vi "Configure Width Trigger.vi"(0 "VISA resource name":refnum<visa-resource-name>, 1 "Trigger Slope (0: Rising)":u16(ring) items=["Rising", "Falling"], 2 "Trigger Source (0: Channel 1)":u16(ring) items=["Channel 1", "Channel 2", "Channel 3", "Channel 4", "External", "Pattern", "Ext", "Ext10"], 5 "Trigger Level (0.0 V)":dbl, 9 "Mode (0: Less Than)":u16(ring) items=["Less Than", "Greater Than", "In Range/Out Of Range"], 11 "error in (no error)":errorcluster, 12 "Limit 1 (4 ns)":dbl=4e-09, 13 "Limit 2 (6 ns)":dbl=6e-09) -> (4 "VISA resource name out":refnum<visa-resource-name>, 15 "error out":errorcluster)   [LabVIEW 2020, in "LeCroy Wave Series.lvlib"]
doc: "Configures width trigger settings. Width trigger allows you to define a positive- or\nnegative-going pulse width bounded by a voltage level, above or below which a trigger\nwill occur. Or you can specify a pulse width and voltage range, within or outside of\nwhich a trigger will occur.\n\nNote: \"External\" is included for the purpose of backwards compatibility. Use EXT or EXT10 for best results."
uses:
  LeCroy Wave Series.lvlib
panel:
  # "Note: \"External\" is included for the purpose\nof backwards compatibility.  Use EXT or EXT10\nfor best results."
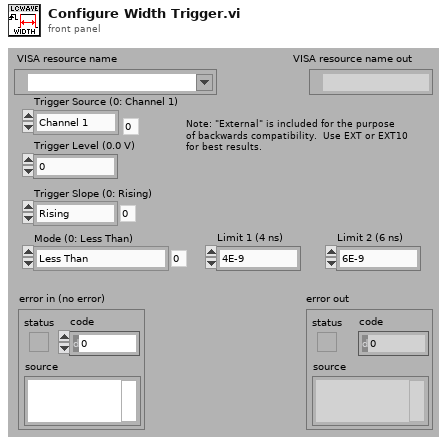
[diagram p1: front panel]
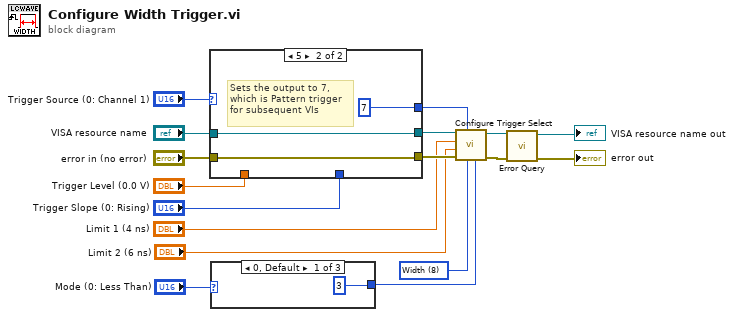
[diagram p0: block diagram]
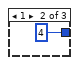
[diagram p2: hidden frame]
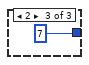
[diagram p3: hidden frame]
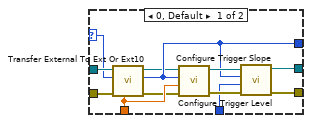
[diagram p4: hidden frame]
diagram:
  w2 = u16 8 items=["Edge", "Dropout", "Glitch", "Interval", "Std", "Sng", "State Qualify", "Edge Qualify", "Width"] ("Trigger type")
  n1 = case shown="5" "Trigger Source (0: Channel 1)" {
    selector: "Trigger Source (0: Channel 1)" -> [w18 _]
    tunnel: "VISA resource name" -> [w22 w32]
    tunnel: "error in (no error)" -> [w23 w31]
    tunnel: "Trigger Level (0.0 V)" -> [w21 _]
    tunnel: "Trigger Slope (0: Rising)" -> [w27 _]
    tunnel: [w26 w32] -> w13
    tunnel: [w25 w31] -> w12
    tunnel: [w24 7] -> w1
    frame 0, Default {
      n2 = call "Transfer External To Ext Or Ext10.vi"("Trigger Level"=w21, "error in (no error)"=w23, "Trigger Source With External"=w18, "VISA resource name"=w22) -> ("error out"=w20:errorcluster, "Trigger Source With Ext/Ext10"=w24:u16, "VISA resource name out"=w19:refnum<visa-resource-name>)  [unwired: 5 in]
      n3 = call "Configure Trigger Level.vi"("error in (no error)"=w20, "Trigger Level 1 (0.0 V)"=w21, "Channel (0: Channel 1)"=w24, "VISA resource name"=w19) -> ("error out"=w28:errorcluster, "VISA resource name out"=w29:refnum<visa-resource-name>)  [unwired: 6 in]
      n4 = call "Configure Trigger Slope.vi"("error in (no error)"=w28, "Trigger Slope (0: Rising)"=w27, "Channel (0: Channel 1)"=w24, "VISA resource name"=w29) -> ("error out"=w25:errorcluster, "VISA resource name out"=w26:refnum<visa-resource-name>)  [unwired: 6 in]
    }
    frame 5 {
      # "Sets the output to 7,\nwhich is Pattern trigger\nfor subsequent VIs"
    }
  }
  n5 = case shown="0, Default" "Mode (0: Less Than)" {
    tunnel: [3 4 7] -> w8
    frame 0, Default {
    }
    frame 1 {
    }
    frame 2 {
    }
  }
  n6 = call "Configure Trigger Select.vi"("Hold Type (0: TI)"=w8, "Trigger type"=w2, "Trigger Source (0: Channel 1)"=w1, "error in (no error)"=w12, "Hold Value 2 (6 ns)"="Limit 2 (6 ns)", "Hold Value 1 (4 ns)"="Limit 1 (4 ns)", "VISA resource name"=w13) -> ("error out"=w4:errorcluster, "VISA resource name out"=w5:refnum<visa-resource-name>)  [unwired: 3 in]
  n7 = call "Error Query.vi"("error in (no error)"=w4, "VISA resource name"=w5) -> ("error out"=→"error out":errorcluster, "VISA resource name out"=→"VISA resource name out":refnum<visa-resource-name>)  [unwired: 6 in, 2 out]
